vi "move_abs.vi"(8 "error in":errorcluster, 10 "Position Aboslute":i32, 11 "VISA in":refnum<visa-resource-name>) -> (0 "error out":errorcluster, 3 "VISA out":refnum<visa-resource-name>)   [LabVIEW 2019]
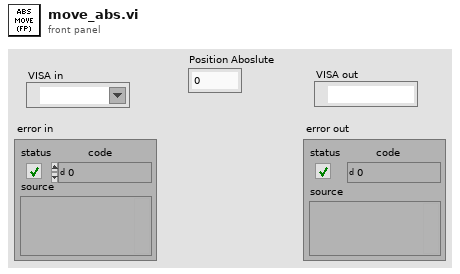
[diagram p1: front panel]
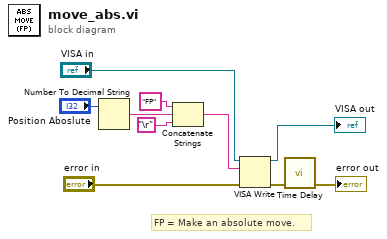
[diagram p0: block diagram]
diagram:
  # "FP = Make an absolute move."
  n1 = Number To Decimal String(number="Position Aboslute") -> (decimal integer string=w4:string)  [unwired: 1 in]
  n2 = Concatenate Strings("FP", w4, "\r") -> (w10:string)
  n3 = VISA Write(VISA resource name="VISA in", write buffer=w10, error in (no error)="error in") -> (VISA resource name out=→"VISA out":refnum<visa-resource-name>, error out=w3:errorcluster)  [unwired: 1 out]
  n4 = call "Time Delay"("error in (no error)"=w3) -> ("error out"=→"error out":errorcluster)  [unwired: 10 in]
